vi "Write scan period (uSec).vi"(8 "error in":errorcluster, 10 "scan period (uSec)":u32=10000, 11 "timing source in":refnum<class "scan engine timing source.lvclass">) -> (0 "error out":errorcluster, 3 "timing source out":refnum<class "scan engine timing source.lvclass">)   [LabVIEW 2013, in "scan engine timing source.lvclass"]
doc: "Sets the configured scan engine period. This configuration is applied by the <b>initialize timing source</b> function. This function sets the <b>set period</b> flag."
uses:
  scan engine timing source.lvclass
  scan engine timing source.lvclass/scan engine timing source.ctl
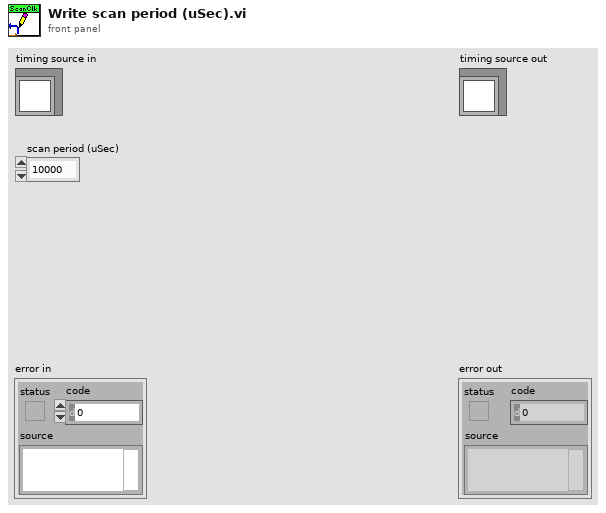
[diagram p1: front panel]
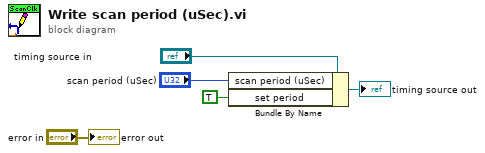
[diagram p0: block diagram]
diagram:
  n1 = Bundle By Name(cluster="timing source in", "scan period (uSec)"="scan period (uSec)", "set period"=TRUE) -> (→"timing source out":refnum<class "scan engine timing source.lvclass">)
  "error out" <- "error in"
